vi "Get Unique Directory.vi"(8 "Error In":errorcluster, 10 "Root Folder Name":string="BeagleBone Black", 11 "Parent Directory":path) -> (0 "Error Out":errorcluster, 3 "Target Directory":path)   [LabVIEW 2020, in "LMH-LINX.lvlib"]
uses:
  LMH-LINX.lvlib
  <vilib>/regexp/Match Regular Expression.xnode
  Toolbox/LMH-Toolbox.lvlib
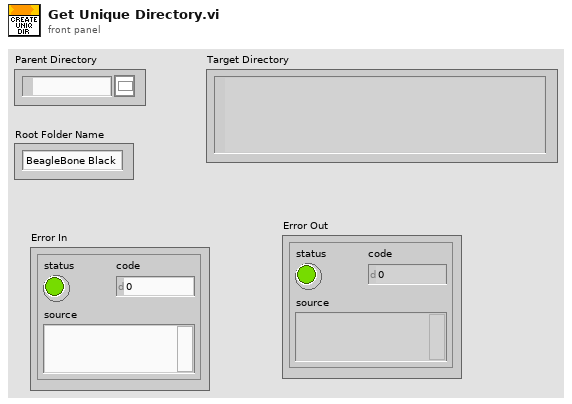
[diagram p1: front panel]
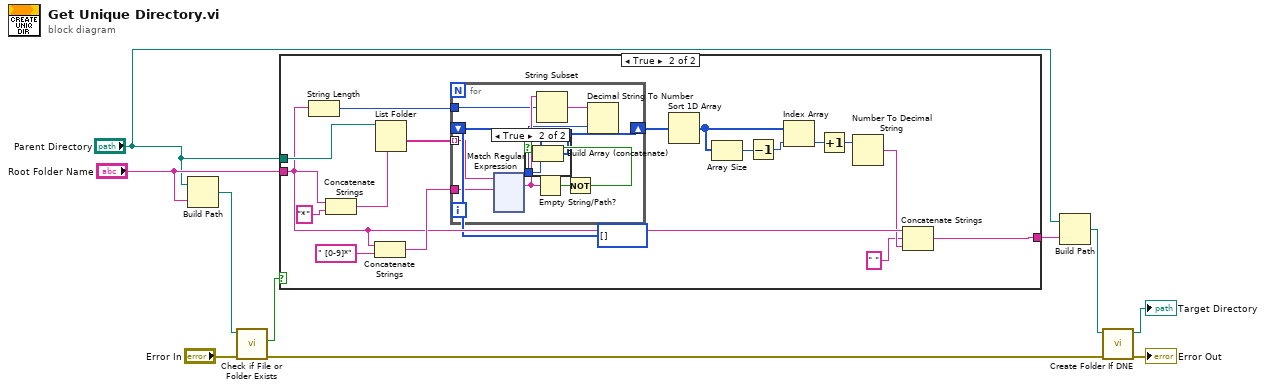
[diagram p0: block diagram]
diagram:
  n1 = Build Path(base path="Parent Directory", name or relative path="Root Folder Name") -> (appended path=w10:path)
  n2 = call <vilib>:"Check if File or Folder Exists.vi"("error in (no error)"="Error In", "path"=w10) -> ("error out"=w3:errorcluster, "file or folder exists?"=w8:bool)  [unwired: 7 in, 1 out]
  n3 = case shown="True" w8 {
    tunnel: [w11 w20] -> w6
    tunnel: "Parent Directory" -> [_ w19]
    tunnel: "Root Folder Name" -> [w11 w17]
    frame False {
    }
    frame True {
      n4 = String Length(string=w17) -> (length=w23:i32)
      n5 = Concatenate Strings(w17, "*" ("string")) -> (w26:string)
      n6 = Concatenate Strings(w17, " [0-9]*" ("string")) -> (w24:string)
      n7 = List Folder(path=w19, pattern=w26) -> (folder names=w22:string[])  [unwired: 1 in, 4 out]
      n8 = for {
        tunnel: w22 -> [w39] mode=indexing
        tunnel: w24 -> [w38]
        tunnel: w23 -> [w35]
        shift-right: [w30] -> w21
        shift-left: i32[] [] ("Array") -> [w31]
        n9 = xnode "Match Regular Expression"("input string"=w39, "regular expression"=w38) -> ("whole match"=w36:string)  [unwired: 4 in, 4 out]
        n10 = Empty String/Path?(string/path=w36) -> (empty?=w37:bool)
        n11 = String Subset(string=w36, offset (0)=w35) -> (substring=w33:string)  [unwired: 1 in]
        n12 = Not(x=w37) -> (.not. x?=w34:bool)
        n13 = Decimal String To Number(string=w33) -> (number=w32:i32)  [unwired: 2 in, 1 out]
        n14 = case shown="True" w34 {
          tunnel: w31 -> [w40 w42]
          tunnel: w32 -> [_ w41]
          tunnel: [w40 w43] -> w30
          frame False {
          }
          frame True {
            n15 = Build Array (concatenate)(w42, w41) -> (w43:i32[])
          }
        }
      }
      n16 = Sort 1D Array(array=w21) -> (sorted array=w14:i32[])
      n17 = Array Size(array=w14) -> (size(s)=w28:i32)
      n18 = Decrement(x=w28) -> (x-1=w27:i32)
      n19 = Index Array(array=w14, index=w27) -> (element=w13:i32)
      n20 = Increment(x=w13) -> (x+1=w18:i32)
      n21 = Number To Decimal String(number=w18) -> (decimal integer string=w16:string)  [unwired: 1 in]
      n22 = Concatenate Strings(w17, " " ("string"), w16) -> (w20:string)
    }
  }
  n23 = Build Path(base path="Parent Directory", name or relative path=w6) -> (appended path=w5:path)
  n24 = call "Create Folder If DNE.vi"("Error In"=w3, "Folder Path"=w5) -> ("Error Out"=→"Error Out":errorcluster, "Dup Path"=→"Target Directory":path)  [unwired: 8 in]
